vi "Acceleration_All_Pulse_Boyer_Mods.vi"() -> ()   [LabVIEW 2015]
uses:
  Control 1 Trigger Source.ctl
  <vilib>/DAQmx/read.llb/DAQmx Read (Analog 1D Wfm NChan NSamp).vi
  <vilib>/DAQmx/create/channels.llb/DAQmx Create Channel (AI-Voltage-Basic).vi
  <vilib>/DAQmx/configure/timing.llb/DAQmx Timing (Sample Clock).vi
  <vilib>/DAQmx/miscellaneous.llb/DAQmx Fill In Error Info.vi
  <vilib>/Waveform/WDTOps.llb/WDT Append Waveforms DBL.vi
  <vilib>/measure/mascope.llb/Pulse Measurements 1 chan.vi
  <vilib>/measure/NI_MAPro.lvlib
panel:
  out "Waveform":waveform(dbl)(graph)
  out "Speed":dbl[](array[numeric])
  out "Period":dbl[](array[numeric])
  out "Boolean":bool
  in  "Tab Control":enum32{"Page 1", "Page 2", "Page 3"}(tab)
  out "Waveform Graph":waveform(dbl)(graph)
  out "Waveform Graph 2":waveform(dbl)(graph)
  out "Waveform Chart 2":dbl(graph)
  out "Waveform Chart":dbl(graph)
  out "data":waveform(dbl)
  out "RPM 2":dbl format="%.2f"
  in  "stop":bool
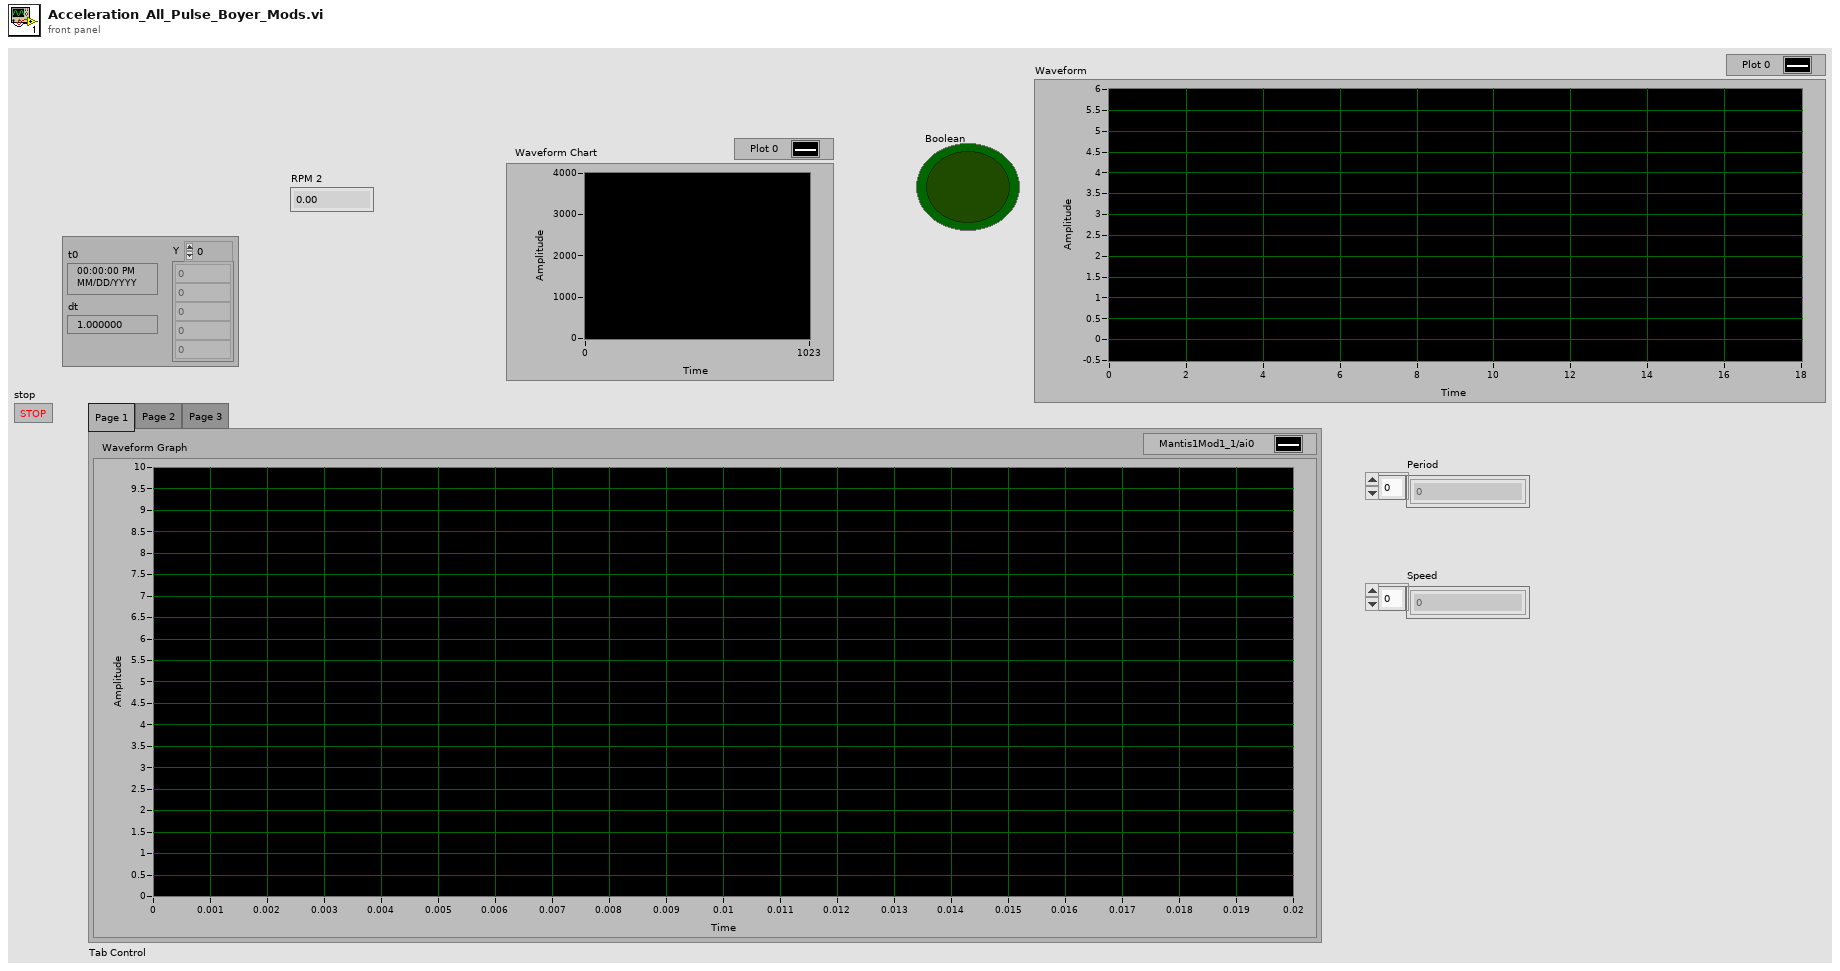
[diagram p1: front panel]
types:
  T1 = typedef "Control 1 Trigger Source.ctl" = cluster{"E-Stop":waveform(dbl), "Stop":waveform(dbl)}
  T2 = cluster{"high ref level":dbl, "mid ref level":dbl, "low ref level":dbl, "ref units":u16}
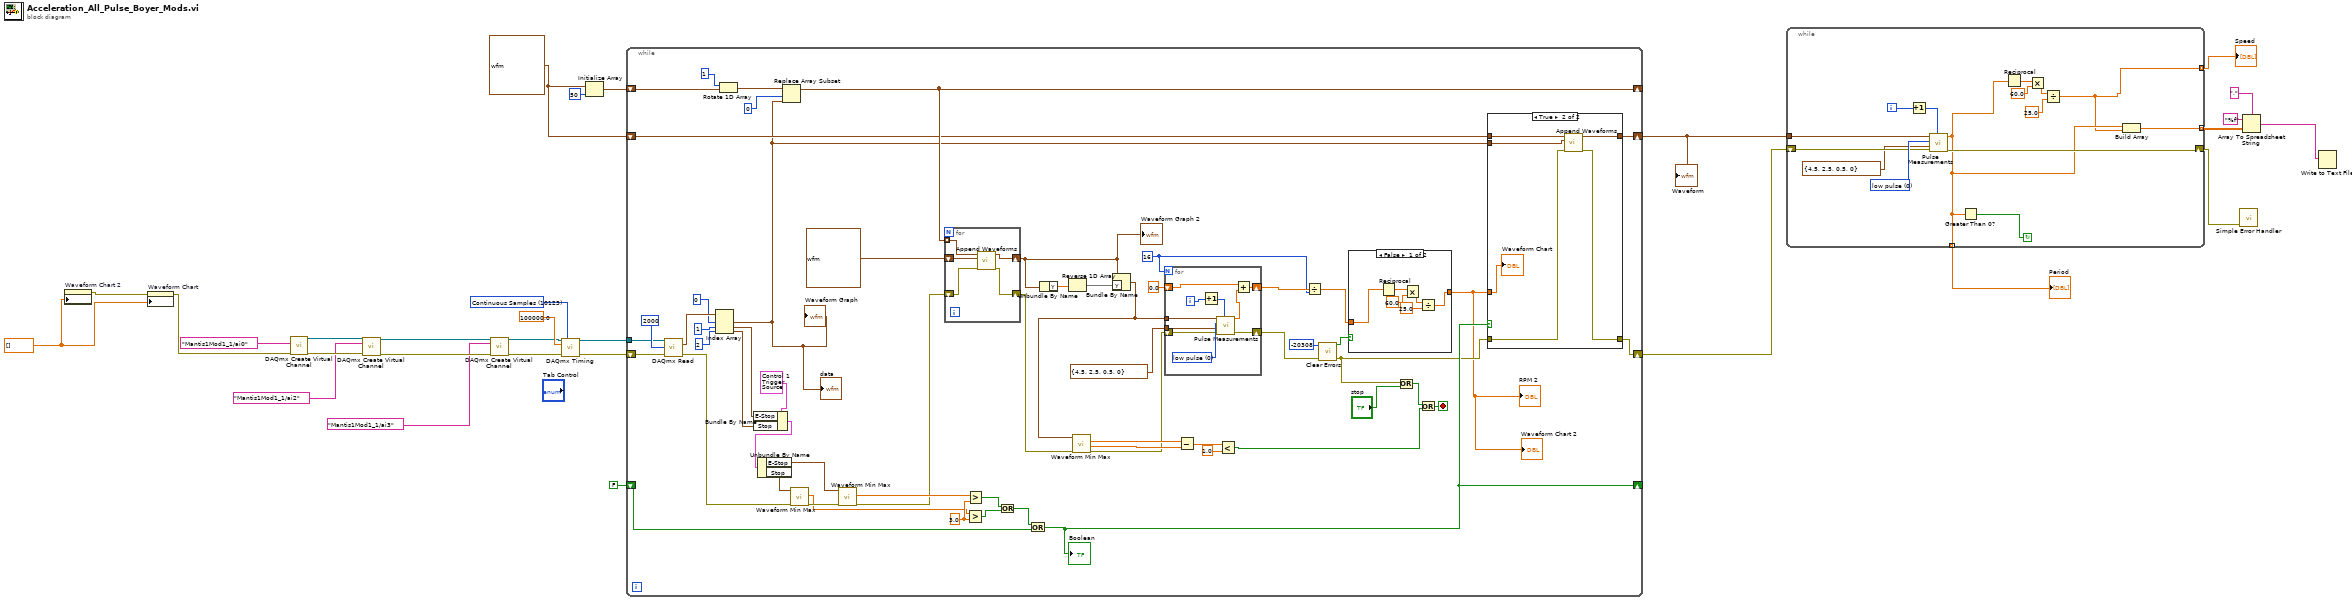
[diagram p0: block diagram]
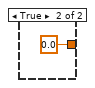
[diagram p3: hidden frame]
diagram:
  w1 = dbl[] [] ("History Data")
  w13 = waveform(dbl) {"t0"=timestamp(0 s since 1904-01-01), "dt"=1e-05, "Y"=[]} ("Waveform")
  w27 = 10123 items=["Finite Samples"=10178, "Continuous Samples"=10123, "Hardware Timed Single Point"=12522] ("sample mode")
  n1 = property on="Waveform Chart 2" class="WFChart (strict)"("History Data"=w1) -> (error out=w2:errorcluster)  [unwired: 2 in, 1 out]
  n2 = property on="Waveform Chart" class="WFChart (strict)"(error in=w2, "History Data"=w1) -> (error out=w10:errorcluster)  [unwired: 1 in, 1 out]
  n3 = call-poly <vilib>:"DAQmx Create Virtual Channel.vi"("physical channels"=tag "Mantis1Mod1_1/ai0", "error in"=w10) -> ("task out"=w22:refnum<k21>, "error out"=w21:errorcluster)  [unwired: 12 in]
  n4 = call-poly <vilib>:"DAQmx Create Virtual Channel.vi"("task in"=w22, "physical channels"=tag "Mantis1Mod1_1/ai2", "error in"=w21) -> ("task out"=w19:refnum<k21>, "error out"=w18:errorcluster)  [unwired: 11 in]
  n5 = call-poly <vilib>:"DAQmx Create Virtual Channel.vi"("task in"=w19, "physical channels"=tag "Mantis1Mod1_1/ai3", "error in"=w18) -> ("task out"=w16:refnum<k21>, "error out"=w17:errorcluster)  [unwired: 11 in]
  n6 = call-poly <vilib>:"DAQmx Timing.vi"("task/channels in"=w16, "sample mode"=w27, "rate"=100000.0, "error in"=w17) -> ("task out"=w26:refnum<k21>, "error out"=w25:errorcluster)  [unwired: 10 in]
  n7 = Initialize Array(w13, 50 ("dimension size")) -> (w23:waveform(dbl)[])
  n8 = while {
    tunnel: w26 -> [w86]
    shift-right: [w80] -> _
    shift-left: w23 -> [w84]
    shift-right: [w35] -> w12
    shift-left: w25 -> [w85]
    shift-right: [w66] -> _
    shift-left: FALSE -> [w70]
    shift-right: [w34] -> w11
    shift-left: w13 -> [w33]
    stop <- w44 stop-if-true
    w63 = 16
    w53 = 3.0 ("y")
    n9 = call-poly <vilib>:"DAQmx Read.vi"("task/channels in"=w86, "number of samples per channel"=2000, "error in"=w85) -> ("data"=w74:waveform(dbl)[], "error out"=w71:errorcluster)  [unwired: 10 in, 1 out]
    n10 = Index Array(array=w74, index #1=0 ("index"), index #2=1 ("index"), index #3=2 ("index")) -> (element #1=w32:waveform(dbl), element #2=w60:waveform(dbl), element #3=w59:waveform(dbl))
    "Waveform Graph" <- w32
    "data" <- w32
    n11 = Rotate 1D Array(1:w84, 2:1 ("n")) -> (0:w82:waveform(dbl)[])
    n12 = Bundle By Name(cluster=T1 {"E-Stop"={"t0"=timestamp(0 s since 1904-01-01), "dt"=1.0, "Y"=[]}, "Stop"={"t0"=timestamp(0 s since 1904-01-01), "dt"=1.0, "Y"=[]}}, "E-Stop"=w60, "Stop"=w59) -> (w54:T1)
    n13 = Unbundle By Name(w54) -> ("E-Stop"=w56:waveform(dbl), "Stop"=w57:waveform(dbl))
    n14 = Replace Array Subset(array=w82, new element=w32, index=0) -> (w80:waveform(dbl)[])
    n15 = call <vilib>:"Waveform Min Max.vi"("error in (no error)"=w71, "waveform in"=w57) -> ("error out"=w58:errorcluster, "Y max"=w52:dbl)  [unwired: 4 in, 4 out]
    n16 = call <vilib>:"Waveform Min Max.vi"("error in (no error)"=w58, "waveform in"=w56) -> ("error out"=w40:errorcluster, "Y max"=w51:dbl)  [unwired: 4 in, 4 out]
    n17 = for {
      tunnel: w80 -> [w115] mode=indexing
      shift-right: [w114] -> w39
      shift-left: w40 -> [w116]
      shift-right: [w113] -> w37
      shift-left: waveform(dbl) {"t0"=timestamp(0 s since 1904-01-01), "dt"=1e-05, "Y"=[]} ("Waveform") -> [w117]
      n18 = call-poly <vilib>:"Append Waveforms.vi"("error in (no error)"=w116, "waveform B"=w117, "waveform A"=w115) -> ("error out"=w114:errorcluster, "waveform out"=w113:waveform(dbl))  [unwired: 7 in]
    }
    "Waveform Graph 2" <- w37
    n19 = Greater?(x=w52, y=w53) -> (0:w49:bool)
    n20 = Greater?(x=w51, y=w53) -> (0:w50:bool)
    n21 = Or(x=w50, y=w49) -> (x .or. y?=w48:bool)
    n22 = Or(x=w48, y=w70) -> (x .or. y?=w66:bool)
    "Boolean" <- w66
    n23 = Unbundle By Name(w37) -> ("Y"=w68:dbl[])
    n24 = Reverse 1D Array(array=w68) -> (reversed array=w67:dbl[])
    n25 = Bundle By Name(cluster=w37, "Y"=w67) -> (w31:waveform(dbl))
    n26 = call <vilib>:"Waveform Min Max.vi"("error in (no error)"=w39, "waveform in"=w31) -> ("error out"=w38:errorcluster, "Y min"=w46:dbl, "Y max"=w47:dbl)  [unwired: 4 in, 3 out]
    n27 = for {
      N: w63 -> [_]
      tunnel: T2 {"high ref level"=4.5, "mid ref level"=2.5, "low ref level"=0.5, "ref units"=0} ("reference levels") -> [w95]
      tunnel: w31 -> [w93]
      shift-right: [w96] -> w79
      shift-left: w38 -> [w94]
      shift-right: [w90] -> w64
      shift-left: 0.0 ("period") -> [w89]
      i -> [w92]
      w97 = u16 0 items=["low pulse", "high pulse"] ("polarity (high)")
      n28 = Increment(x=w92) -> (x+1=w91:i32)
      n29 = call-poly <vilib>:"Pulse Measurements.vi"("pulse number (1)"=w91, "error in (no error)"=w94, "reference levels"=w95, "polarity (high)"=w97, "signal in"=w93) -> ("error out"=w96:errorcluster, "period"=w88:dbl)  [unwired: 2 in, 3 out]
      n30 = Add(x=w89, y=w88) -> (x+y=w90:dbl)
    }
    n31 = Subtract(x=w47, y=w46) -> (x-y=w43:dbl)
    n32 = Less?(x=w43, y=1.0) -> (x < y?=w41:bool)
    n33 = Divide(x=w64, y=w63) -> (x/y=w62:dbl)
    n34 = call <vilib>:"Clear Errors.vi"("error in (no error)"=w79, "specific error code to clear (0: all)"=-20308) -> ("error out"=w36:errorcluster, "specific error cleared?"=w77:bool)  [unwired: 4 in]
    n35 = case shown="False" w77 {
      tunnel: w62 -> [w111 _]
      tunnel: [w108 0.0] -> w30
      frame False {
        n36 = Reciprocal(x=w111) -> (1/x=w109:dbl)
        n37 = Multiply(x=w109, y=60.0) -> (x*y=w107:dbl)
        n38 = Divide(x=w107, y=25.0) -> (x/y=w108:dbl)
      }
      frame True {
      }
    }
    "RPM 2" <- w30
    "Waveform Chart 2" <- w30
    n39 = Or(x=w36, y="stop") -> (x .or. y?=w45:bool)
    n40 = Or(x=w45, y=w41) -> (x .or. y?=w44:bool)
    n41 = case shown="True" w66 {
      tunnel: w30 -> [_ w105]
      tunnel: w36 -> [w99 w102]
      tunnel: [w99 w101] -> w35
      tunnel: [w98 w103] -> w34
      tunnel: w33 -> [w98 w104]
      tunnel: w32 -> [_ w100]
      frame False {
      }
      frame True {
        n42 = call-poly <vilib>:"Append Waveforms.vi"("error in (no error)"=w102, "waveform B"=w100, "waveform A"=w104) -> ("error out"=w101:errorcluster, "waveform out"=w103:waveform(dbl))  [unwired: 7 in]
        "Waveform Chart" <- w105
      }
    }
  }
  "Waveform" <- w11
  n43 = while {
    tunnel: w11 -> [w131]
    shift-right: [w126] -> w3
    shift-left: w12 -> [w130]
    tunnel: [w120] -> w9 mode=indexing
    tunnel: [w119] -> w8 mode=indexing
    tunnel: [w118] -> w6 mode=indexing
    i -> [w128]
    stop <- w125 continue-if-true
    w132 = u16 0 items=["low pulse", "high pulse"] ("polarity (high)")
    n44 = Increment(x=w128) -> (x+1=w127:i32)
    n45 = call-poly <vilib>:"Pulse Measurements.vi"("pulse number (1)"=w127, "error in (no error)"=w130, "reference levels"=T2 {"high ref level"=4.5, "mid ref level"=2.5, "low ref level"=0.5, "ref units"=0}, "polarity (high)"=w132, "signal in"=w131) -> ("error out"=w126:errorcluster, "period"=w120:dbl)  [unwired: 2 in, 3 out]
    n46 = Greater Than 0?(x=w120) -> (x > 0?=w125:bool)
    n47 = Reciprocal(x=w120) -> (1/x=w123:dbl)
    n48 = Multiply(x=w123, y=60.0) -> (x*y=w122:dbl)
    n49 = Divide(x=w122, y=25.0) -> (x/y=w119:dbl)
    n50 = Build Array(w120, w119) -> (w118:dbl[])
  }
  "Period" <- w9
  "Speed" <- w8
  n51 = call <vilib>:"Simple Error Handler.vi"("error in (no error)"=w3) -> ()  [unwired: 4 in, 5 out]
  n52 = Array To Spreadsheet String(delimiter (Tab)=",", array=w6, 3:"%f" ("format string")) -> (spreadsheet string=w5:string)
  n53 = Write to Text File(text=w5) -> ()  [unwired: 3 in, 3 out]
